vi "Test DAQmx Bus Multisample Analog Input.vi"() -> ()   [LabVIEW 2021]
uses:
  <vilib>/TSA/Omni-Bus/Omni-Bus/Omni_Bus.lvclass
  <vilib>/TSA/Omni-Bus/Omni-Bus/Support/Broad Types.ctl
  <vilib>/Utility/Data Type/Type Definitions/Data Type.ctl
  <vilib>/TSA/Abstract Data Classes/Abs_Types/Type/Abs_Type.lvclass/Abs_Type.ctl
  <vilib>/TSA/Omni-Bus/Omni-Bus/Omni_Bus.lvclass/Omni_Bus.ctl
  <vilib>/TSA/Omni-Bus/Omni-Bus/Support/Read/Read Multi Waveform.vi
  <vilib>/TSA/Omni-Bus/Omni-Bus/Support/Read/Read Waveform.vi
  <vilib>/TSA/Omni-Bus/Omni-Bus/Support/Get/Get Multi Waveform.vi
  <vilib>/TSA/Omni-Bus/Omni-Bus/Support/FindVar.vi
  <vilib>/TSA/Omni-Bus/Omni-Bus/Support/FindMultiVar.vi
  <vilib>/Utility/error.llb/Clear Errors.vi
  <vilib>/TSA/Omni-Bus/Omni-Bus/Properties/Read Var Map.vi
  <vilib>/TSA/Abstract Data Classes/Abs_Types/Type/Properties/Read Tag.vi
  Source/DAQmx-Bus.lvclass
  C:/Program Files (x86)/National Instruments/LabVIEW 2021/vi.lib/TSA/Omni-Bus/Omni-Bus/Bus Access/Bus_Access.lvclass
  <vilib>/TSA/Abstract Data Classes/Abs_Types/Waveform/Abs_Waveform.lvclass
  C:/Program Files (x86)/National Instruments/LabVIEW 2021/vi.lib/TSA/Abstract Data Classes/Abs_Types/Type/Abs_Type.lvclass
  <vilib>/TSA/Abstract Data Classes/Abs_Types/Value/Abs_Value.lvclass
  <vilib>/TSA/Omni-Bus/Omni-Bus/Support/Check For Read Only Error.vi
  <vilib>/TSA/Omni-Bus/Omni-Bus/Support/Incorrect Tag String Error.vi
  <vilib>/TSA/Abstract Data Classes/Abs_Types/Type/Abs_Type.lvclass
  <vilib>/Utility/Data Type/NI_Data Type.lvlib
panel:
  out "Waveform Graph":waveform(dbl)[](graph)
  out "Numeric":i32
  out "Waveform Chart":waveform(dbl)(graph)
  out "timed out?":bool
  in  "stop":bool
  in  "Combo Box":string(combo)
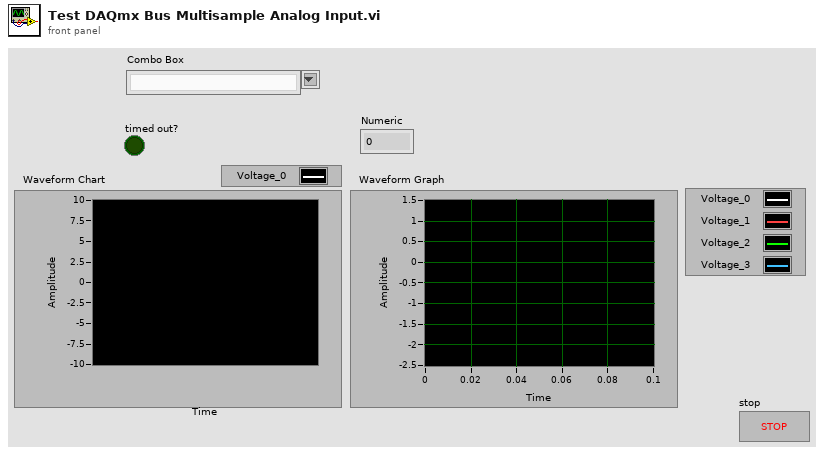
[diagram p1: front panel]
types:
  T1 = typedef "NI_Data Type.lvlib/Data Type.ctl" = enum8{"Invalid Type", "Void", "I8", "I16", "I32", "I64", "U8", "U16", "U32", "U64", "Single Float", "Double Float", "Extended Float", "Single Complex", "Double Complex", "Extended Complex", "Enum U8", "Enum U16", "Enum U32", "Enum U64", "Single Float With Unit", "Double Float With Unit", "Extended Float With Unit", "Single Complex with Unit", "Double Complex with Unit", "Extended Complex with Unit", "Boolean", "String", "Path", "Picture", "Tag", "Array", "Cluster", "Variant", "LV Variant", "Waveform", "Timestamp", "Digital Waveform", "Digital Data", "ExpressData", "Refnum", "External Data", "VI", "Poly VI", "LabVIEW Class Instance", "Fixed Point", "Set Collection", "Map Collection"}
  T2 = typedef "Omni_Bus.lvclass/Broad Types.ctl" = enum16{"All Tags", "NI Specific Type", "Boolean", "String", "Numeric", "Float", "Integer", "Collection", "All Value Types", "Non Value Types"}
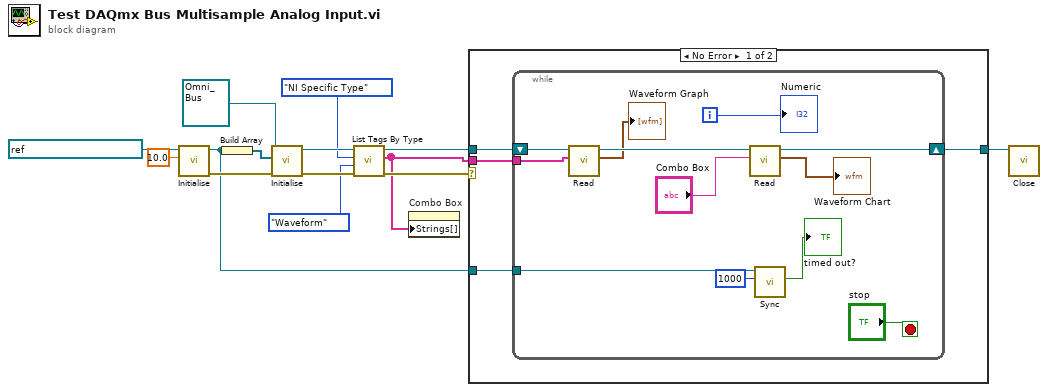
[diagram p0: block diagram]
diagram:
  n1 = call "Initialise.vi"("timeout (s)"=10.0 ("timeout"), "DAQmx Device"=refnum<k21> "MultisampleVoltage") -> ("error out"=w10:errorcluster, "DAQmx-Bus out"=w3:refnum<class "DAQmx-Bus.lvclass">)  [unwired: 8 in]
  n2 = Build Array(w3) -> (w12:refnum<class "DAQmx-Bus.lvclass">[])
  n3 = call-dynamic "Initialise.vi"("error in (no error)"=w10, "Bus Access"=w12, "Var Bus in"=refnum<class "Omni_Bus.lvclass"> refnum) -> ("error out"=w7:errorcluster, "Var Bus out"=w8:refnum<class "Omni_Bus.lvclass">)  [unwired: 7 in]
  n4 = call <vilib>:"List Tags By Type.vi"("error in (no error)"=w7, "NI Specific Type"=Data_Type."Waveform", "Broad Types"=Broad_Types."NI Specific Type", "Var Bus in"=w8) -> ("error out"=w5:errorcluster, "Tags"=w1:string[], "Var Bus out"=w6:refnum<class "Omni_Bus.lvclass">)  [unwired: 4 in, 1 out]
  n5 = property on="Combo Box" class="CmbBox"("Strings[]"=w1) -> ()  [unwired: 2 in, 2 out]
  n6 = case shown="No Error" w5 {
    tunnel: [w18 w31] -> w9
    tunnel: w6 -> [w17 w31]
    tunnel: w3 -> [w16 _]
    tunnel: w1 -> [w15 _]
    frame No Error {
      n7 = while {
        shift-right: [w30] -> w18
        shift-left: w17 -> [w22]
        tunnel: w16 -> [w27]
        tunnel: w15 -> [w21]
        i -> [w23]
        stop <- "stop" stop-if-true
        n8 = call-poly <vilib>:"Read.vi"("Tag"=w21, "Var Bus in"=w22) -> ("Waveform"=→"Waveform Graph":waveform(dbl)[], "Var Bus out"=w20:refnum<class "Omni_Bus.lvclass">)  [unwired: 7 in, 1 out]
        n9 = call-poly <vilib>:"Read.vi"("Tag"="Combo Box", "Var Bus in"=w20) -> ("Waveform"=→"Waveform Chart":waveform(dbl), "Var Bus out"=w30:refnum<class "Omni_Bus.lvclass">)  [unwired: 7 in, 1 out]
        n10 = call-dynamic "Sync.vi"("timeout in ms (-1)"=1000, "DAQmx-Bus in"=w27) -> ("timed out?"=→"timed out?":bool)  [unwired: 7 in, 2 out]
        "Numeric" <- w23
      }
    }
    frame Error {
    }
  }
  n11 = call-dynamic "Close.vi"("Data in"=w9) -> ()  [unwired: 9 in, 2 out]
